vi "ASI Get Gain Offset.vi"(6 "Offset_LowestRN":i32, 7 "Gain_LowestRN":i32, 9 "Offset_UnityGain":i32, 10 "Offset_HighestDR":i32, 11 "iCameraID":i32) -> (1 "Offset_UnityGain out":i32, 2 "Offset_HighestDR out":i32, 3 "function return":i32, 4 "Offset_LowestRN out":i32, 5 "Gain_LowestRN out":i32)   [LabVIEW 2012, in "ASICamera2_no_err.lvlib"]
doc: "ASICAMERA_API ASI_ERROR_CODE ASIGetGainOffset(int iCameraID, int *Offset_HighestDR, int *Offset_UnityGain, int *Gain_LowestRN, int *Offset_LowestRN);"
uses:
  <userlib>/ASICamera2_no_err/ASICamera2_no_err.lvlib
  <userlib>/ASICamera2_no_err/ASICamera2.dll
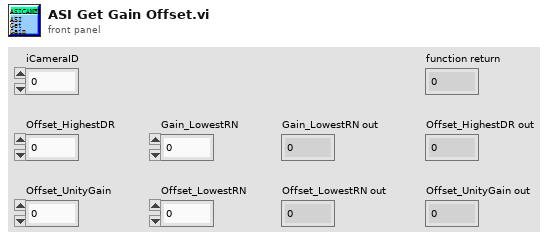
[diagram p1: front panel]
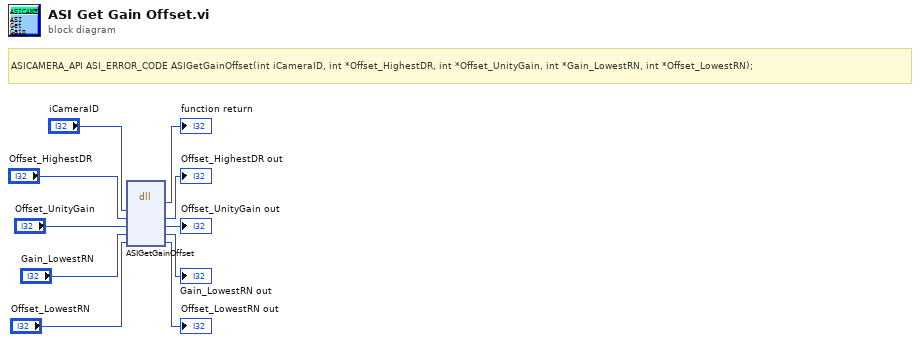
[diagram p0: block diagram]
diagram:
  # "ASICAMERA_API ASI_ERROR_CODE ASIGetGainOffset(int iCameraID, int *Offset_HighestDR, int *Offset_UnityGain, int *Gain_LowestRN, int *Offset_LowestRN);"
  n1 = dll-call lib="D:/Program Files (x86)/National Instruments/LabVIEW 2012/user.lib/ASICamera2_no_err/ASICamera2.*" fn="ASIGetGainOffset"("iCameraID"="iCameraID", "Offset_HighestDR"="Offset_HighestDR", "Offset_UnityGain"="Offset_UnityGain", "Gain_LowestRN"="Gain_LowestRN", "Offset_LowestRN"="Offset_LowestRN") -> (→"function return":i32, "Offset_HighestDR"=→"Offset_HighestDR out":i32, "Offset_UnityGain"=→"Offset_UnityGain out":i32, "Gain_LowestRN"=→"Gain_LowestRN out":i32, "Offset_LowestRN"=→"Offset_LowestRN out":i32)  [unwired: 4 in, 2 out]
